vi "DIAG_STM Get Meta Data.vi"   [LabVIEW 2015, in "Diagnostics Addon Engine.lvlib"]
doc: "Returns the meta data associated with the STM session."
uses:
  Diagnostics Addon Engine.lvlib
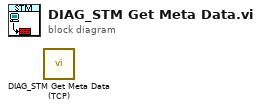
[diagram p0: block diagram]
diagram:
  n1 = call "DIAG_STM Get Meta Data (TCP).vi"() -> ()  [unwired: 9 in, 3 out]
